vi "Temp Setpoint Limits--SubVI.vi"(4 "Instance(1)":i32=1, 6 "Limits":T2={"Upper Limit"=175.0, "Lower Limit"=-73.0}, 7 "Temp Units":T1=enum."Degrees C", 8 "error in (no error)":errorcluster, 10 "Get/Set":enum16{"Get", "Set"}(ring), 11 "Watlow F4T in":refnum<class "Watlow F4T.lvclass">) -> (0 "error out":errorcluster, 3 "Watlow F4T out":refnum<class "Watlow F4T.lvclass">)   [LabVIEW 2024, in "Watlow F4T.lvclass"]
uses:
  Watlow F4T.lvclass
  Process Controller/Controls/Limits--Cluster.ctl
  Process Controller/Controls/Temperature Units--Enum.ctl
  Controls/Standard Bus Commands--Enum.ctl
  Watlow F4T.lvclass/Watlow F4T.ctl
  Process Controller/_Thermal Process Controller.lvclass
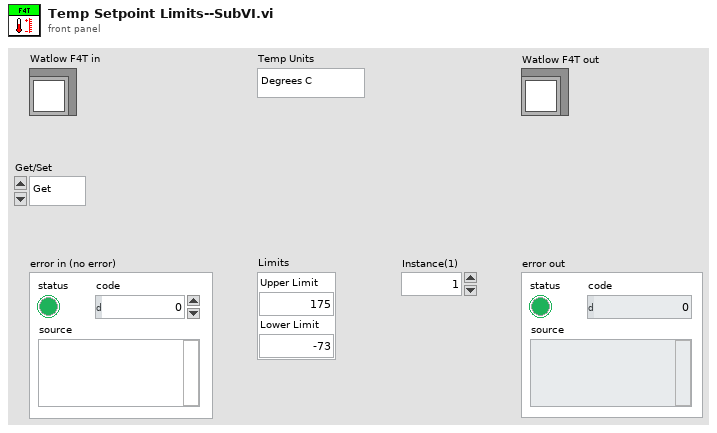
[diagram p1: front panel]
types:
  T1 = typedef "_Thermal Process Controller.lvclass/Temperature Units--Enum.ctl" = enum16{"Degrees F", "Degrees C", "Degrees K"}
  T2 = typedef "_Thermal Process Controller.lvclass/Limits--Cluster.ctl" = cluster{"Upper Limit":dbl, "Lower Limit":dbl}
  T3 = typedef "Watlow F4T.lvclass/Standard Bus Commands--Enum.ctl" = enum16{"Remote Setpoint", "Remote Mode", "Temp Feedback", "Target Setpoint", "Current Setpoint", "Setpoint Lower Limit", "Setpoint Upper Limit", "Ramp Rate Y", "Ramp Rate X", "Ramp Rate Action", "Temp Control State", "Temp Control Mode", "Power", "Heat Power", "Cool Power"}
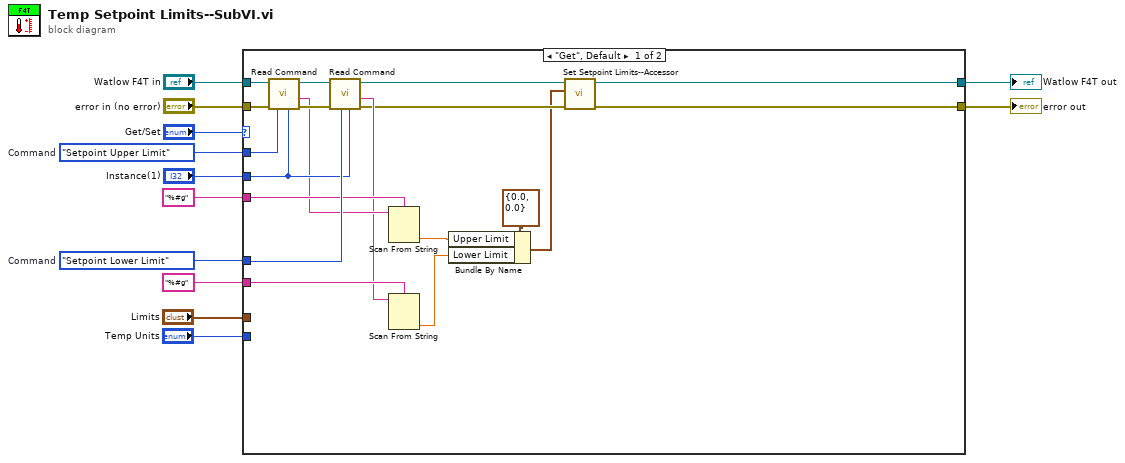
[diagram p0: block diagram]
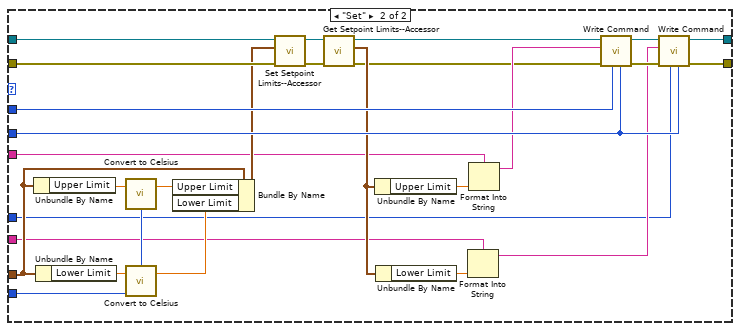
[diagram p2: hidden frame]
diagram:
  w3 = Standard_Bus_Commands--Enum."Setpoint Lower Limit"  # Command
  w8 = Standard_Bus_Commands--Enum."Setpoint Upper Limit"  # Command
  n1 = case shown="\"Get\", Default" "Get/Set" {
    tunnel: [w14 w58] -> w12
    tunnel: "%#g" ("format string") -> [w24 w37]
    tunnel: "Instance(1)" -> [w25 w54]
    tunnel: w8 -> [w31 w55]
    tunnel: [w13 w53] -> w7
    tunnel: "Watlow F4T in" -> [w30 w52]
    tunnel: "error in (no error)" -> [w29 w49]
    tunnel: "%#g" ("format string") -> [w23 w38]
    tunnel: w3 -> [w26 w34]
    tunnel: "Limits" -> [_ w45]
    tunnel: "Temp Units" -> [_ w47]
    frame "Get", Default {
      n2 = call "Read Command.vi"("Instance"=w25, "Commands"=w31, "error in (no error)"=w29, "Watlow F4T In"=w30) -> ("error out"=w28:errorcluster, "Value Out"=w19:string, "Watlow F4T out"=w27:refnum<class "Watlow F4T.lvclass">)  [unwired: 5 in]
      n3 = call "Read Command.vi"("Instance"=w25, "Commands"=w26, "error in (no error)"=w28, "Watlow F4T In"=w27) -> ("error out"=w17:errorcluster, "Value Out"=w18:string, "Watlow F4T out"=w16:refnum<class "Watlow F4T.lvclass">)  [unwired: 5 in]
      n4 = Scan From String(format string=w24, input string=w19) -> (output 1=w21:dbl)  [unwired: 3 in, 3 out]
      n5 = Scan From String(format string=w23, input string=w18) -> (output 1=w20:dbl)  [unwired: 3 in, 3 out]
      n6 = Bundle By Name(cluster=T2 {"Upper Limit"=0.0, "Lower Limit"=0.0} ("Limits"), "Upper Limit"=w21, "Lower Limit"=w20) -> (w15:T2)
      n7 = call "Set Setpoint Limits--Accessor.vi"("error in (no error)"=w17, "Limits"=w15, "Watlow F4T in"=w16) -> ("error out"=w14:errorcluster, "Watlow F4T out"=w13:refnum<class "Watlow F4T.lvclass">)  [unwired: 7 in]
    }
    frame "Set" {
      n8 = Unbundle By Name(w45) -> ("Upper Limit"=w48:dbl)
      n9 = Unbundle By Name(w45) -> ("Lower Limit"=w46:dbl)
      n10 = call "Convert to Celsius.vi"("Temp In"=w48, "Temp Units"=w47) -> ("Temp Out"=w44:dbl)  [unwired: 3 in]
      n11 = call "Convert to Celsius.vi"("Temp In"=w46, "Temp Units"=w47) -> ("Temp Out"=w43:dbl)  [unwired: 3 in]
      n12 = Bundle By Name(cluster=w45, "Upper Limit"=w44, "Lower Limit"=w43) -> (w42:T2)
      n13 = call "Set Setpoint Limits--Accessor.vi"("error in (no error)"=w49, "Limits"=w42, "Watlow F4T in"=w52) -> ("error out"=w50:errorcluster, "Watlow F4T out"=w51:refnum<class "Watlow F4T.lvclass">)  [unwired: 7 in]
      n14 = call "Get Setpoint Limits--Accessor.vi"("error in (no error)"=w50, "Watlow F4T in"=w51) -> ("error out"=w32:errorcluster, "Limits"=w41:T2, "Watlow F4T out"=w33:refnum<class "Watlow F4T.lvclass">)  [unwired: 7 in]
      n15 = Unbundle By Name(w41) -> ("Upper Limit"=w40:dbl)
      n16 = Unbundle By Name(w41) -> ("Lower Limit"=w39:dbl)
      n17 = Format Into String(format string=w38, w39) -> (resulting string=w35:string)  [unwired: 2 in, 1 out]
      n18 = Format Into String(format string=w37, w40) -> (resulting string=w36:string)  [unwired: 2 in, 1 out]
      n19 = call "Write Command.vi"("Instance"=w54, "Commands"=w55, "error in (no error)"=w32, "Set Value"=w36, "Watlow F4T In"=w33) -> ("error out"=w56:errorcluster, "Watlow F4T out"=w57:refnum<class "Watlow F4T.lvclass">)  [unwired: 5 in]
      n20 = call "Write Command.vi"("Instance"=w54, "Commands"=w34, "error in (no error)"=w56, "Set Value"=w35, "Watlow F4T In"=w57) -> ("error out"=w58:errorcluster, "Watlow F4T out"=w53:refnum<class "Watlow F4T.lvclass">)  [unwired: 5 in]
    }
  }
  "error out" <- w12
  "Watlow F4T out" <- w7
